vi "Set IED stop notifier.vi"(10 "IED Notifier":refnum<notifier>, 11 "IED in":refnum<class "IED.lvclass">) -> (3 "IED out":refnum<class "IED.lvclass">)   [LabVIEW 2015, in "IED Actor.lvlib" / "IED.lvclass"]
uses:
  IED.lvclass
  IED.lvclass/IED.ctl
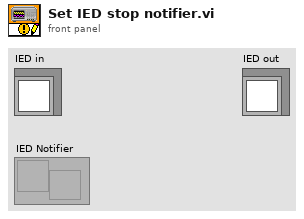
[diagram p1: front panel]
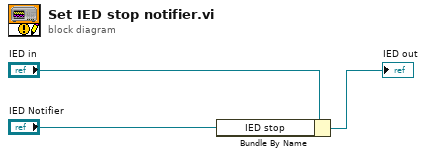
[diagram p0: block diagram]
diagram:
  n1 = Bundle By Name(cluster="IED in", "IED stop"="IED Notifier") -> (→"IED out":refnum<class "IED.lvclass">)
